vi "ULx Write (Composite 2D  NChan NSamp).vi"(0 "task in":refnum<k24>, 1 "auto start":bool, 5 "analog data":dbl[][](array[numeric]), 7 "digital data":u32[][](array[numeric]) format="%#.0f", 9 "timeout":dbl=10.0 format="%_4g", 11 "error in":errorcluster) -> (4 "task out":refnum<k24>, 10 "number of samples written per channel":u32, 15 "error out":errorcluster)   [LabVIEW 2020]
doc: "Writes one or more samples to a composite output task that contains that contains one or more analog output channels."
uses:
  C:/Users/William/Documents/LV 2020 builds/LeaktestDAQ/Source-v33/ULx_LV.dll
  ULx_LV.dll
panel:
  # "channel"
  # "sample #"
  # "channel"
  # "sample #"
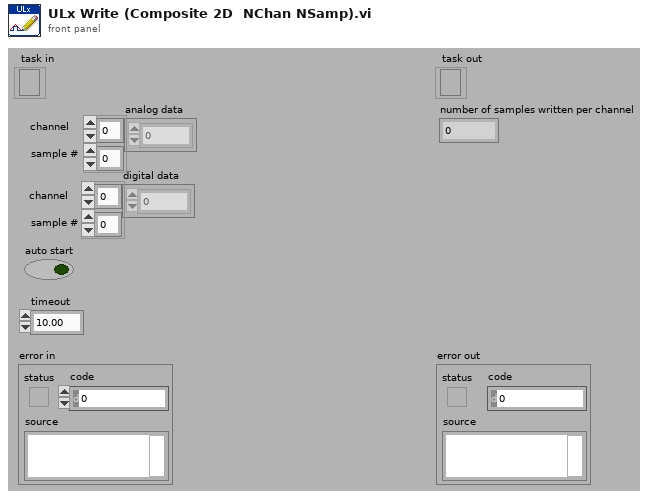
[diagram p1: front panel]
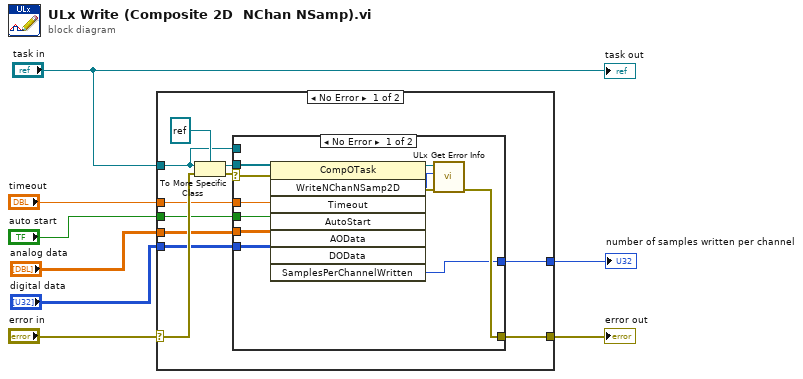
[diagram p0: block diagram]
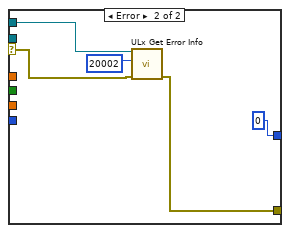
[diagram p2: hidden frame]
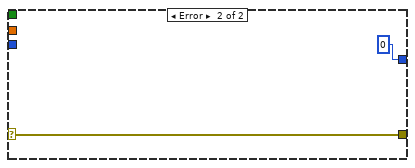
[diagram p3: hidden frame]
diagram:
  n1 = case shown="No Error" "error in" {
    selector: "error in" -> [w19 w37]
    tunnel: "task in" -> [w13 _]
    tunnel: "timeout" -> [w15 _]
    tunnel: [w14 w37] -> w6
    tunnel: "auto start" -> [w12 _]
    tunnel: [w11 0 ("SamplesPerChannelWritten")] -> w3
    tunnel: "analog data" -> [w10 _]
    tunnel: "digital data" -> [w9 _]
    frame No Error {
      n2 = To More Specific Class(target class=refnum<k24> refnum, reference=w13, error in=w19) -> (specific class reference=w16:refnum<k24>, error out=w17:errorcluster)
      n3 = case shown="No Error" w17 {
        selector: w17 -> [w29 w31]
        tunnel: w16 -> [w30 _]
        tunnel: w15 -> [w24 _]
        tunnel: [w26 w34] -> w14
        tunnel: w13 -> [_ w33]
        tunnel: w10 -> [w22 _]
        tunnel: w12 -> [w23 _]
        tunnel: [w21 0 ("SamplesPerChannelWritten")] -> w11
        tunnel: w9 -> [w20 _]
        frame No Error {
          n4 = invoke class="CompOTask" method="WriteNChanNSamp2D"(reference=w30, error in=w29, "Timeout"=w24, "AutoStart"=w23, "AOData"=w22, "DOData"=w20) -> (reference out=w27:refnum<k24>, error out=w28:errorcluster, "WriteNChanNSamp2D"=w25:i32, "SamplesPerChannelWritten"=w21:u32)  [unwired: 2 in, 4 out]
          n5 = call "ULx Get Error Info.vi"("error in"=w28, "ErrorCode"=w25, "task in"=w27) -> ("error out"=w26:errorcluster)  [unwired: 8 in]
        }
        frame Error {
          n6 = call "ULx Get Error Info.vi"("error in"=w31, "ErrorCode"=20002, "task in"=w33) -> ("error out"=w34:errorcluster)  [unwired: 8 in]
        }
      }
    }
    frame Error {
    }
  }
  "error out" <- w6
  "number of samples written per channel" <- w3
  "task out" <- "task in"
